vi "Data_base_server.vi"(0 "Raw Data Pathname":path, 1 "Results File Pathname":path, 3 "Clients time":dbl, 4 "Start time":dbl, 5 "End time":dbl, 6 "Average Meas Time (min)":dbl=100.0 format="%.1f", 7 "Channels from Client":string[][](array[string])=[["Data Base:Measurement:Type", "LDA & Cw"], ["Data Base:Position:No of Inst", "2"], ["Data Base:Position:X1", "-60"], ["Data Base:Position:X2", ""], ["Data Base:Position:Y1", "2"], ["Data Base:Position:Y2", "0.00"], ["Data Base:Position:Z1", "0.00"], ["Data Base:Position:Z2", "2.00"]], 8 "Average Sampling freq":sgl=100.0 format="%.1f", 9 "Rig Name":string) -> (14 "Channel names":string[](array[string])=["Data Base:DB:Filename", "Data Base:Start:Date", "Data Base:Start:Time", "EnFlo Tun:Job: Name", "EnFlo Tun:User: Name", "Data Base:Results:Folder", "Data Base:Results:Filename", "Data Base:Measurement:Type", "Data Base:X Axis:Max", "Data Base:X Axis:Min", "Data Base:Y Axis:Max", "Data Base:Y Axis:Min", "Data Base:Z Axis:Max", "Data Base:Z Axis:Min", "Data Base:No of:Measurements", "Data Base:Av Meas:Frequency (Hz)", "Data Base:Av Meas:Time (min)", "EnFlo Tun:labstrat1:Delta T", "EnFlo Tun:Heater Temp:Average", "EnFlo Tun:Inside:Velocity", "EnFlo Tun:Vorticity: Generators", "EnFlo Tun:Barrier Wall: Height", "EnFlo Tun:Roughness: Height", "EnFlo Tun:Side Wall: Separation", "EnFlo Tun:Obstacle/:Building", "EnFlo Tun:Obstacle: Orientation", "GMU:Source: Type", "GMU:Source: Height", "GMU:Release: Orientation", "GMU:Source:Meas Q", "GMU:Source:Meas Strength", "GMU:Trace: Gas", "GMU:Carrier: Gas", "GMU:Source:Release Temp", "GMU:Suction:Meas Q"], 15 "Channel values":string[](array[string])=["1999:May_1999:G3_3 HD_00006", "13/5/99", "1:55 pm", "National Power", "Paul Hayden", "BMT", "default", "LDA, Cw", "100.00", "-60.00", "2.00", "0.00", "0.00", "0.00", "10", "100.00", "100.00", "1.42", "26.63", "1.54", "\"7 quarter elipticals, 1 metre tall\"", "150mm", "20mm", "No sidewalls installed", "National Power Building", "30 deg", "D=17.5mm", "150 mm", "Vertical", "", "", "Ethane", "48% N2 in He", "", ""], 17 "spreadsheet string":string)   [LabVIEW 2012]
doc: "This is an example of using features of the VI Server as a client. It shows how you might browse from one or more applications that may be exporting data from one or more data stations. \n\nThe example shows how to query a server for its list of exported VIs, how to get references to the VIs, and how call them with the Call By Reference function."
uses:
  ADAM_Global.vi
  Sub VI's/Exp conditions/EnFlo_Tun_Setup_global.vi
  Anemometry/Anemometry Sub Vis/Globals/Constants_global.vi
panel:
  out "Output Array":string[][](array[string])
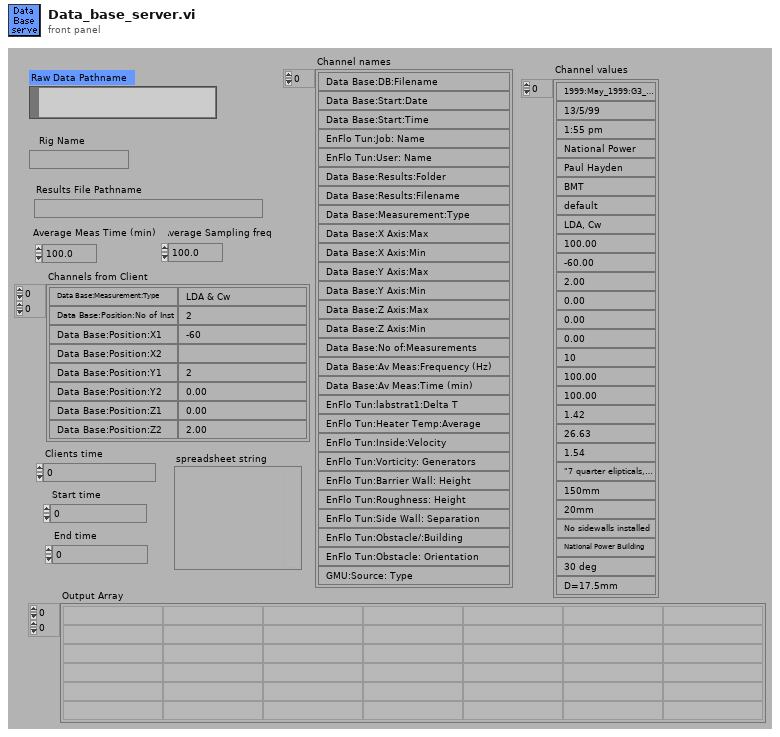
[diagram p1: front panel]
types:
  T1 = cluster{"second":i32, "minute":i32, "hour":i32, "day of month":i32, "month":i32, "year":i32, "day of week":i32, "day of year":i32, "is DST":i32}
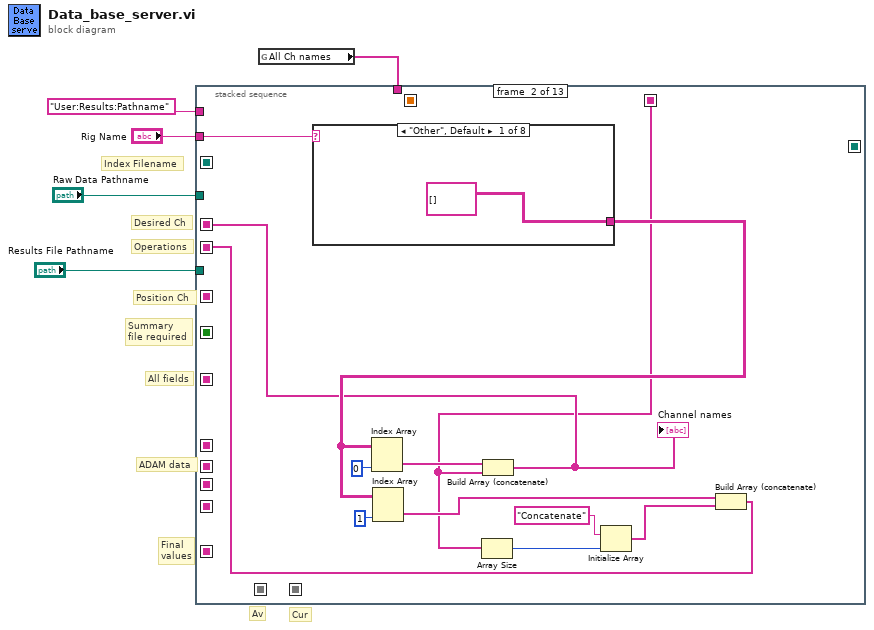
[diagram p0: block diagram]
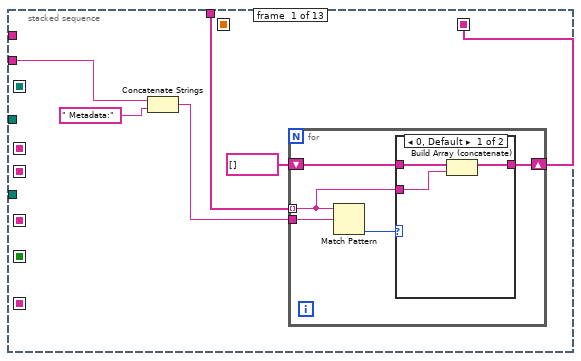
[diagram p2: hidden frame]
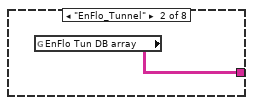
[diagram p4: hidden frame]
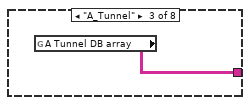
[diagram p5: hidden frame]
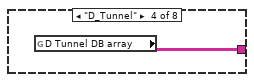
[diagram p6: hidden frame]
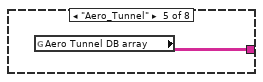
[diagram p7: hidden frame]
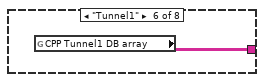
[diagram p8: hidden frame]
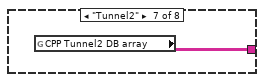
[diagram p9: hidden frame]
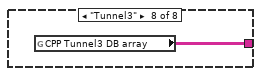
[diagram p10: hidden frame]
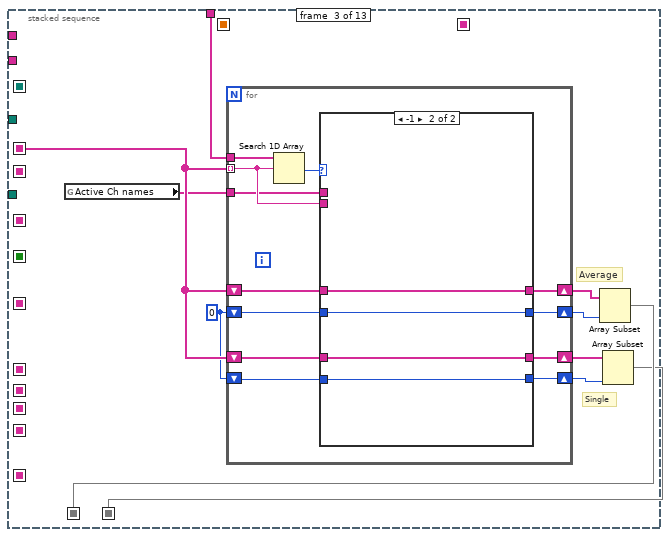
[diagram p11: hidden frame]
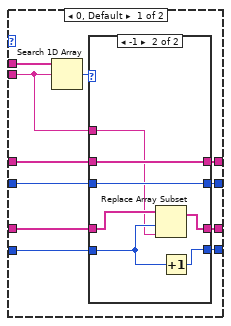
[diagram p12: hidden frame]
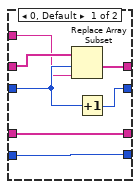
[diagram p13: hidden frame]
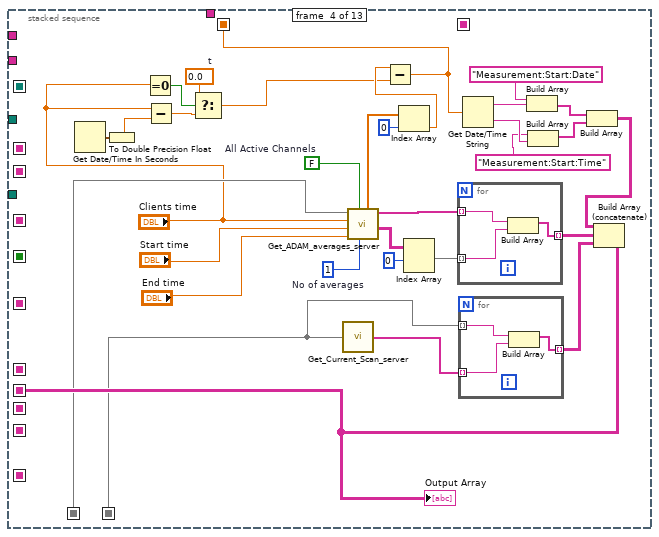
[diagram p14: hidden frame]
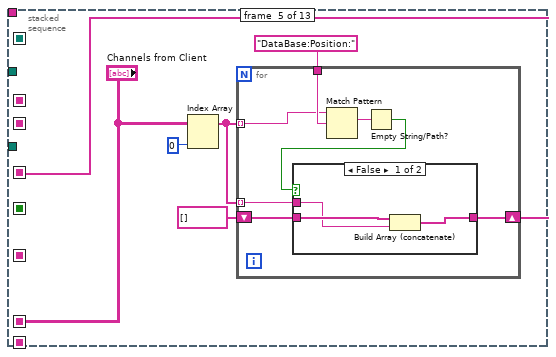
[diagram p15: hidden frame]
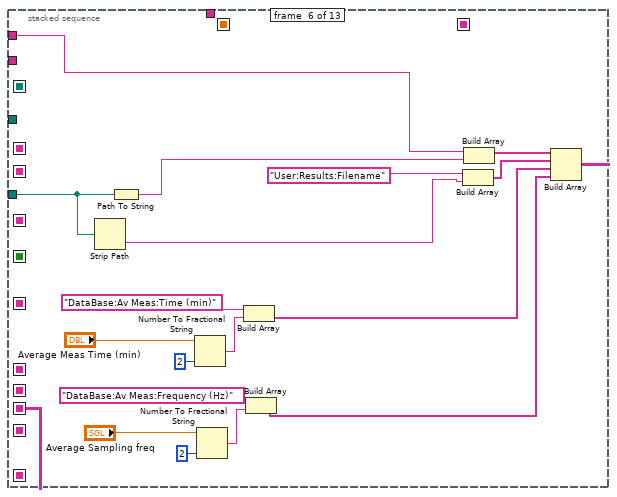
[diagram p17: hidden frame]
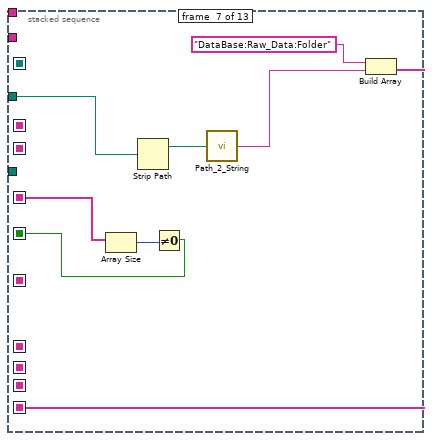
[diagram p18: hidden frame]
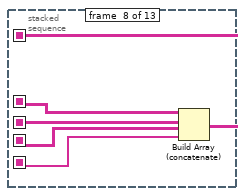
[diagram p19: hidden frame]
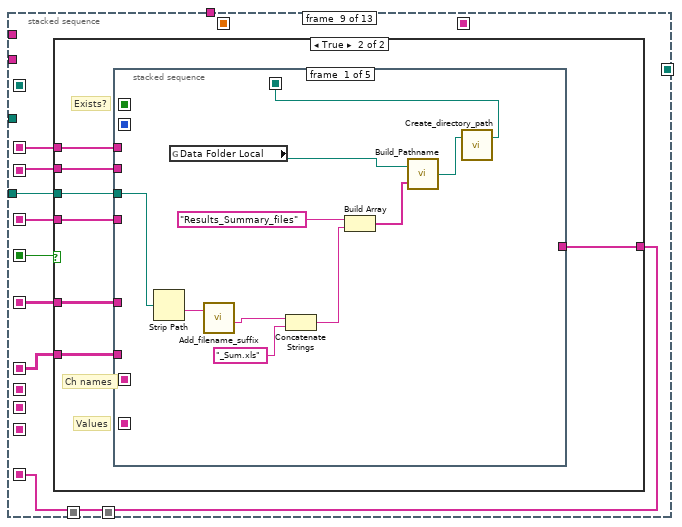
[diagram p20: hidden frame]
diagram:
  # "Cur"
  # "Av"
  # "Index Filename"
  # "Desired Ch"
  # "Operations"
  # "Final\nvalues"
  # "Summary\nfile required"
  # "Position Ch"
  # "All fields"
  # "ADAM data"
  n1 = global read "ADAM_Global.vi" "All Ch names"() -> (w3:string[])
  n2 = stacked-sequence {
    seq-local: [_ w27 _ _ _ _ _ _ _ _ _ _ _] -> [_ _ w50 _ _ _ _ _ w183 _ _ w319 w331]
    seq-local: [_ _ _ w112 _ _ _ _ _ _ _ _ _] -> [_ _ _ _ _ _ _ w177 _ _ _ _ _]
    seq-local: [_ _ _ _ _ w164 _ _ _ _ _ _ _] -> [_ _ _ _ _ _ _ w176 _ _ _ _ _]
    seq-local: [_ _ _ _ _ _ _ w173 _ _ _ _ _] -> [_ _ _ _ _ _ _ _ w181 w280 _ _ _]
    seq-local: [_ _ _ _ _ _ w168 _ _ _ _ _ _] -> [_ _ _ _ _ _ _ w175 _ _ _ _ _]
    seq-local: [_ _ _ _ _ _ _ _ w185 _ _ _ _] -> [_ _ _ _ _ _ _ _ _ w287 _ w320 w330]
    seq-local: [_ _ _ _ w131 _ _ _ _ _ _ _ _] -> [_ _ _ _ _ _ w171 _ w182 _ _ _ _]
    seq-local: [_ _ _ _ "Channels from Client" _ _ _ _ _ _ _ _] -> [_ _ _ _ _ _ _ w174 w178 _ _ _ _]
    seq-local: [_ _ _ _ _ _ w169 _ _ _ _ _ _] -> [_ _ _ _ _ _ _ _ w184 _ _ _ _]
    seq-local: [_ w21 _ _ _ _ _ _ _ _ _ _ _] -> [_ _ _ _ _ _ _ _ w180 _ _ _ _]
    seq-local: [_ _ _ w93 _ _ _ _ _ _ _ _ _] -> [_ _ _ _ _ _ _ _ _ _ _ _ _]
    seq-local: [_ _ _ _ _ _ _ _ _ _ w305 _ _] -> [_ _ _ _ _ _ _ _ _ _ _ w317 w323]
    seq-local: [_ _ w43 _ _ _ _ _ _ _ _ _ _] -> [_ _ _ w104 _ _ _ _ _ _ _ _ _]
    seq-local: [_ _ w42 _ _ _ _ _ _ _ _ _ _] -> [_ _ _ w103 _ _ _ _ _ _ _ _ _]
    seq-local: [w6 _ _ _ _ _ _ _ _ _ _ _ _] -> [_ w24 _ _ _ _ _ _ _ _ _ _ _]
    seq-local: [_ _ _ _ _ _ _ _ _ _ w307 _ _] -> [_ _ _ _ _ _ _ _ _ _ _ _ w322]
    tunnel: "User:Results:Pathname" -> [_ _ _ _ _ w152 _ _ _ _ _ w321 _]
    tunnel: "Results File Pathname" -> [_ _ _ _ _ w149 _ _ w179 _ _ _ _]
    tunnel: "Rig Name" -> [w10 w29 _ _ _ _ _ _ _ w273 w314 _ _]
    tunnel: w3 -> [w8 _ w41 _ _ _ _ _ _ _ _ _ _]
    tunnel: "Raw Data Pathname" -> [_ _ _ _ _ _ w167 _ _ _ _ _ _]
    frame #0 {
      n3 = Concatenate Strings(w10, " Metadata:") -> (w9:string)
      n4 = for {
        tunnel: w9 -> [w13]
        shift-right: [w14] -> w6
        shift-left: string[] [] -> [w15]
        tunnel: w8 -> [w12] mode=indexing
        n5 = Match Pattern(string=w12, regular expression=w13) -> (offset past match=w16:i32)  [unwired: 4 out]
        n6 = case shown="0, Default" w16 {
          tunnel: w15 -> [w19 w20]
          tunnel: [w17 w20] -> w14
          tunnel: w12 -> [w18 _]
          frame 0, Default {
            n7 = Build Array (concatenate)(w19, w18) -> (w17:string[])
          }
          frame -1 {
          }
        }
      }
    }
    frame #1 {
      n8 = case shown="\"Other\", Default" w29 {
        tunnel: [string[][] [] ("EnFlo Tun DB array") w34 w35 w36 w37 w38 w39 w40] -> w30
        frame "Other", Default {
        }
        frame "EnFlo_Tunnel" {
          n9 = global read "EnFlo_Tun_Setup_global.vi" "EnFlo Tun DB array"() -> (w34:string[][])
        }
        frame "A_Tunnel" {
          n10 = global read "EnFlo_Tun_Setup_global.vi" "A Tunnel DB array"() -> (w35:string[][])
        }
        frame "D_Tunnel" {
          n11 = global read "EnFlo_Tun_Setup_global.vi" "D Tunnel DB array"() -> (w36:string[][])
        }
        frame "Aero_Tunnel" {
          n12 = global read "EnFlo_Tun_Setup_global.vi" "Aero Tunnel DB array"() -> (w37:string[][])
        }
        frame "Tunnel1" {
          n13 = global read "EnFlo_Tun_Setup_global.vi" "CPP Tunnel1 DB array"() -> (w38:string[][])
        }
        frame "Tunnel2" {
          n14 = global read "EnFlo_Tun_Setup_global.vi" "CPP Tunnel2 DB array"() -> (w39:string[][])
        }
        frame "Tunnel3" {
          n15 = global read "EnFlo_Tun_Setup_global.vi" "CPP Tunnel3 DB array"() -> (w40:string[][])
        }
      }
      n16 = Index Array(array=w30, index (col)=0) -> (element=w28:string[])  [unwired: 1 in]
      n17 = Index Array(array=w30, index (col)=1) -> (element=w26:string[])  [unwired: 1 in]
      n18 = Array Size(array=w24) -> (size(s)=w25:i32)
      n19 = Build Array (concatenate)(w28, w24) -> (w27:string[])
      "Channel names" <- w27
      n20 = Initialize Array("Concatenate", w25) -> (w22:string[])
      n21 = Build Array (concatenate)(w26, w22) -> (w21:string[])
    }
    frame #2 {
      w48 = 0
      # "Single"
      # "Average"
      n22 = global read "ADAM_Global.vi" "Active Ch names"() -> (w49:string[])
      n23 = for {
        tunnel: w50 -> [w56] mode=indexing
        tunnel: w41 -> [w62]
        shift-right: [w60] -> w47
        shift-left: w50 -> [w59]
        shift-right: [w58] -> w45
        shift-left: w50 -> [w57]
        tunnel: w49 -> [w55]
        shift-right: [w51] -> w46
        shift-left: w48 -> [w52]
        shift-right: [w53] -> w44
        shift-left: w48 -> [w54]
        n24 = Search 1D Array(1D array=w62, element=w56) -> (index of element=w61:i32)  [unwired: 1 out]
        n25 = case shown="-1" w61 {
          tunnel: [w64 w91] -> w60
          tunnel: w59 -> [w65 w91]
          tunnel: [w70 w90] -> w58
          tunnel: w57 -> [w71 w90]
          tunnel: w56 -> [w63 _]
          tunnel: w55 -> [w73 _]
          tunnel: w54 -> [w69 w88]
          tunnel: [w68 w88] -> w53
          tunnel: w52 -> [w67 w89]
          tunnel: [w66 w89] -> w51
          frame 0, Default {
            n26 = Search 1D Array(1D array=w73, element=w63) -> (index of element=w72:i32)  [unwired: 1 out]
            n27 = case shown="-1" w72 {
              tunnel: w71 -> [w76 w87]
              tunnel: [w76 w86] -> w70
              tunnel: w69 -> [w75 w85]
              tunnel: [w75 w84] -> w68
              tunnel: w67 -> [w80 w83]
              tunnel: [w77 w83] -> w66
              tunnel: w65 -> [w79 w82]
              tunnel: [w78 w82] -> w64
              tunnel: w63 -> [w74 w81]
              frame 0, Default {
                n28 = Replace Array Subset(array=w79, new element=w74, index=w80) -> (w78:string[])
                n29 = Increment(x=w80) -> (x+1=w77:i32)
              }
              frame -1 {
                n30 = Replace Array Subset(array=w87, new element=w81, index=w85) -> (w86:string[])
                n31 = Increment(x=w85) -> (x+1=w84:i32)
              }
            }
          }
          frame -1 {
          }
        }
      }
      n32 = Array Subset(array=w47, length=w46) -> (w43:string[])  [unwired: 1 in]
      n33 = Array Subset(array=w45, length=w44) -> (w42:string[])  [unwired: 1 in]
    }
    frame #3 {
      w97 = 0.0  # t
      w105 = FALSE  # All Active Channels
      w123 = 1  # No of averages
      n34 = Get Date/Time In Seconds() -> (seconds since 1Jan1904=w92:timestamp)
      n35 = To Double Precision Float(number=w92) -> (double precision float=w100:dbl)
      n36 = Equal To 0?(x="Clients time") -> (x = 0?=w98:bool)
      n37 = Subtract(x="Clients time", y=w100) -> (x-y=w99:dbl)
      n38 = Select(t=w97, s=w98, f=w99) -> (s? t:f=w94:dbl)
      n39 = call "Get_Current_Scan_server.vi"("Desired Channels"=w103) -> ("String values"=w102:string[])  [unwired: 2 out]
      n40 = call "Get_ADAM_averages_server.vi"("No of averages"=w123, "All Active Channels"=w105, "End time"="End time", "Start time"="Start time", "Clients time"="Clients time", "ADAM Ch Names"=w104) -> ("Values"=w108:string[][], "Titles"=w111:string[], "Times"=w121:dbl[])  [unwired: 2 out]
      n41 = Index Array(array=w121, index=0) -> (element=w95:dbl)
      n42 = Subtract(x=w95, y=w94) -> (x-y=w93:dbl)
      n43 = Index Array(array=w108, index (row)=0) -> (element=w110:string[])  [unwired: 1 in]
      n44 = for {
        tunnel: w111 -> [w129] mode=indexing
        tunnel: w110 -> [w128] mode=indexing
        tunnel: [w127] -> w113 mode=indexing
        n45 = Build Array(w129, w128) -> (w127:string[])
      }
      n46 = for {
        tunnel: w102 -> [w126] mode=indexing
        tunnel: [w125] -> w101 mode=indexing
        tunnel: w103 -> [w124] mode=indexing
        n47 = Build Array(w124, w126) -> (w125:string[])
      }
      n48 = Get Date/Time String(seconds (now)=w93) -> (date string=w119:string, time string=w118:string)  [unwired: 2 out]
      n49 = Build Array("Measurement:Start:Date", w119) -> (w116:string[])
      n50 = Build Array("Measurement:Start:Time", w118) -> (w115:string[])
      n51 = Build Array(w116, w115) -> (w114:string[][])
      n52 = Build Array (concatenate)(w114, w113, w101) -> (w112:string[][])
      "Output Array" <- w112
    }
    frame #4 {
      n53 = Index Array(array="Channels from Client", index (col)=0) -> (element=w133:string[])  [unwired: 1 in]
      n54 = for {
        tunnel: "DataBase:Position:" ("String to match") -> [w142]
        tunnel: w133 -> [w141] mode=indexing
        shift-right: [w136] -> w131
        shift-left: string[] [] -> [w137]
        tunnel: w133 -> [w138] mode=indexing
        n55 = Match Pattern(string=w141, regular expression=w142) -> (match substring=w140:string)  [unwired: 4 out]
        n56 = Empty String/Path?(string/path=w140) -> (empty?=w139:bool)
        n57 = case shown="False" w139 {
          tunnel: w138 -> [w143 _]
          tunnel: w137 -> [w145 w146]
          tunnel: [w144 w146] -> w136
          frame False {
            n58 = Build Array (concatenate)(w145, w143) -> (w144:string[])
          }
          frame True {
          }
        }
      }
    }
    frame #5 {
      n59 = Strip Path(path=w149) -> (name=w148:string)  [unwired: 1 out]
      n60 = Path To String(path=w149) -> (string=w151:string)
      n61 = Number To Fractional String(number="Average Meas Time (min)", precision (6)=i16 2) -> (F-format string=w161:string)  [unwired: 2 out]
      n62 = Number To Fractional String(number="Average Sampling freq", precision (6)=i16 2) -> (F-format string=w159:string)  [unwired: 2 out]
      n63 = Build Array("DataBase:Av Meas:Time (min)", w161) -> (w155:string[])
      n64 = Build Array("DataBase:Av Meas:Frequency (Hz)", w159) -> (w154:string[])
      n65 = Build Array("User:Results:Filename", w148) -> (w147:string[])
      n66 = Build Array(w152, w151) -> (w153:string[])
      n67 = Build Array(w153, w147, w155, w154) -> (w164:string[][])
    }
    frame #6 {
      n68 = Array Size(array=w171) -> (size(s)=w170:i32)
      n69 = Strip Path(path=w167) -> (stripped path=w166:path)  [unwired: 1 out]
      n70 = Not Equal To 0?(x=w170) -> (x != 0?=w169:bool)
      n71 = call "Path_2_String.vi"("Real Path"=w166) -> ("Path String"=w165:string)
      n72 = Build Array("DataBase:Raw_Data:Folder", w165) -> (w168:string[])
    }
    frame #7 {
      n73 = Build Array (concatenate)(w174, w177, w176, w175) -> (w173:string[][])
    }
    frame #8 {
      n74 = case shown="True" w184 {
        tunnel: [w187 w199] -> w185
        tunnel: w183 -> [w188 w198]
        tunnel: w182 -> [_ w197]
        tunnel: w181 -> [w189 w196]
        tunnel: w180 -> [_ w195]
        tunnel: w179 -> [_ w194]
        tunnel: w178 -> [_ w193]
        frame False {
          n75 = Index Array(array=w189, index (col)=1) -> (element=w190:string[])  [unwired: 1 in]
          n76 = Index Array(array=w189, index (col)=0) -> (element=w186:string[])  [unwired: 1 in]
          n77 = call "Merge_row_values.vi"("Present Row values"=w190, "Present Channels"=w186, "Desired Channels"=w188) -> ("Desired Row values"=w187:string[])  [unwired: 1 out]
        }
        frame True {
          # "Exists?"
          # "Ch names"
          # "Values"
          n78 = stacked-sequence {
            seq-local: [_ _ w230 _ _] -> [_ _ _ w246 w269]
            seq-local: [_ _ w226 _ _] -> [_ _ _ w250 w271]
            seq-local: [w207 _ _ _ _] -> [_ w213 w228 _ w272]
            seq-local: [_ w210 _ _ _] -> [_ _ w222 _ w270]
            seq-local: [_ _ w223 _ _] -> [_ _ _ _ w268]
            tunnel: [_ _ _ w251 _] -> w199
            tunnel: w198 -> [_ _ w229 w248 _]
            tunnel: w197 -> [_ _ w236 _ _]
            tunnel: w196 -> [_ _ w232 _ _]
            tunnel: w195 -> [_ _ _ w249 _]
            tunnel: w194 -> [w208 _ _ _ _]
            tunnel: w193 -> [_ w216 _ _ _]
            frame #0 {
              n79 = Strip Path(path=w208) -> (name=w201:string)  [unwired: 1 out]
              n80 = global read "Constants_global.vi" "Data Folder Local"() -> (w206:path)
              n81 = call "Add_filename_suffix.vi"("Filename"=w201) -> ("Base name"=w200:string)  [unwired: 1 in, 3 out]
              n82 = Concatenate Strings(w200, "_Sum.xls" ("Substring")) -> (w202:string)
              n83 = Build Array("Results_Summary_files", w202) -> (w205:string[])
              n84 = call "Build_Pathname.vi"("PathElements"=w205, "PathnameIn"=w206) -> ("AppendedPath"=w203:path)
              n85 = call "Create_directory_path.vi"("Path name"=w203) -> ("Path name Out"=w207:path)  [unwired: 1 in, 1 out]
            }
            frame #1 {
              n86 = Index Array(array=w216, index (col)=0) -> (element=w220:string[])  [unwired: 1 in]
              n87 = Search 1D Array(1D array=w220, element="Does the results file already exist?") -> (index of element=w217:i32)  [unwired: 1 out]
              n88 = Index Array(array=w216, index (row)=w217, index (col)=1 ("Index")) -> (element=w215:string)
              n89 = call "Does_file_exist_(simple).vi"("Pathname"=w213) -> ("exists?"=w211:bool)
              n90 = Not Equal?(x="FALSE", y=w215) -> (x != y?=w212:bool)
              n91 = And(x=w211, y=w212) -> (x .and. y?=w210:bool)
            }
            frame #2 {
              n92 = Build Array (concatenate)(w229, w236) -> (w235:string[])
              n93 = case shown="True" w222 {
                tunnel: w235 -> [w239 w245]
                tunnel: w228 -> [_ w244]
                tunnel: [w239 w243] -> w226
                tunnel: [string[][] [] ("Channel Values") w242] -> w224
                tunnel: [0 ("Offset from File End") w241] -> w223
                frame False {
                }
                frame True {
                  n94 = call "Read_Ch_data_file.vi"("Present Channels"=w245, "Output"=enum16{"All Ch data", "The last few rows"}."All Ch data", "Filename"=w244) -> ("Channel Values"=w242:string[][], "Merged Channels"=w243:string[], "Offset from File End"=w241:i32)  [unwired: 2 in, 2 out]
                }
              }
              n95 = Index Array(array=w232, index (col)=1) -> (element=w231:string[])  [unwired: 1 in]
              n96 = Index Array(array=w232, index (col)=0) -> (element=w227:string[])  [unwired: 1 in]
              n97 = call "Merge_row_values.vi"("Present Row values"=w231, "Present Channels"=w227, "Desired Channels"=w226) -> ("Desired Row values"=w225:string[])  [unwired: 1 out]
              n98 = Build Array (concatenate)(w224, w225) -> (w230:string[][])
            }
            frame #3 {
              n99 = call "Average_Column_Values.vi"("Present Values"=w246, "Present Channels"=w250, "Channel operations"=w249, "Channel names for operations"=w248) -> ("Desired Row values"=w247:string[])
              n100 = call "String_to_Pos_array.vi"("Channel values"=w246, "Channel names"=w250) -> ("Positions"=w254:dbl[][], "No of Inst"=w253:i32)
              n101 = while {
                tunnel: [w260] -> w252
                tunnel: w253 -> [w264]
                tunnel: w254 -> [w259]
                i -> [w257]
                stop <- w261 continue-if-true
                w255 = 3 ("x")
                n102 = Increment(x=w257) -> (x+1=w265:i32)
                n103 = Multiply(x=w255, y=w257) -> (x*y=w256:i32)
                n104 = Array Subset(array=w259, index (col)=w256, length (col)=w255) -> (w258:dbl[][])  [unwired: 2 in]
                n105 = call "Cal_Pos_Max_Min.vi"("Positions"=w258) -> ("Position Info"=w260:string[][], "Instrument moved?"=w262:bool)
                n106 = Less?(x=w265, y=w264) -> (x < y?=w263:bool)
                n107 = Compound Arithmetic op=AND(invert w262, w263) -> (w261:bool)
              }
              n108 = call "Replace_Channel_Values.vi"("Channels to replace"=w252, "Present Values"=w247, "Present Channels"=w248) -> ("Merged Row values"=w251:string[])  [unwired: 1 out]
            }
            frame #4 {
              w266 = TRUE  # Lock File
              w267 = TRUE  # Append last row only
              n109 = call "Write_Ch_data_file.vi"("Append last row only"=w267, "Lock File"=w266, "exists?"=w270, "Write offset fr file end"=w268, "Channel Values"=w269, "Channel names"=w271, "Filename"=w272) -> ()  [unwired: 1 in, 4 out]
            }
          }
        }
      }
    }
    frame #9 {
      n110 = Index Array(array=w280, index (col)=0) -> (element=w284:string[])  [unwired: 1 in]
      n111 = Concatenate Strings(w273, ":Pitot:Velocity" ("Substring")) -> (w286:string)
      n112 = Concatenate Strings(w273, ":Speed:Dem Velocity" ("Substring")) -> (w275:string)
      n113 = Concatenate Strings(w273, ":Speed:Calib Tweak" ("Substring")) -> (w274:string)
      n114 = Build Array(w275, w274, w286) -> (w283:string[])
      n115 = for {
        tunnel: w284 -> [w303]
        tunnel: w283 -> [w302] mode=indexing
        tunnel: [w301] -> w282 mode=indexing
        tunnel: [w300] -> w279 mode=indexing
        n116 = Search 1D Array(1D array=w303, element=w302) -> (index of element=w300:i32)  [unwired: 1 out]
        n117 = Greater Or Equal To 0?(x=w300) -> (x >= 0?=w301:bool)
      }
      n118 = And Array Elements(Boolean array=w282) -> (logical AND=w281:bool)
      n119 = case shown="True" w281 {
        tunnel: w280 -> [_ w294]
        tunnel: w279 -> [_ w292]
        tunnel: w273 -> [_ w290]
        frame False {
        }
        frame True {
          w288 = FALSE  # Tunnel Heated?
          n120 = Index Array(array=w294, index (col)=1) -> (element=w293:string[])  [unwired: 1 in]
          n121 = for {
            tunnel: w293 -> [w299]
            tunnel: w292 -> [w298] mode=indexing
            tunnel: [w296] -> w291 mode=indexing
            n122 = Index Array(array=w299, index=w298) -> (element=w297:string)
            n123 = Fract/Exp String To Number(string=w297) -> (number=w296:dbl)  [unwired: 4 out]
          }
          n124 = call "Add_to_speed_calib_file.vi"("New Row"=w291, "Tunnel Heated?"=w288, "Rig Name"=w290, "Mode"=enum16{"Add Row", "Get Error Value"}."Add Row") -> ()  [unwired: 2 in, 2 out]
        }
      }
      "Channel values" <- w287
    }
    frame #10 {
      n125 = Get Date/Time In Seconds() -> (seconds since 1Jan1904=w304:timestamp)
      n126 = global read "Constants_global.vi" "Data Folder Local"() -> (w309:path)
      n127 = call <vilib>:"LV70TimeStampToDateRec.vi"("time stamp"=w304) -> ("date time rec"=w316:T1)
      n128 = global read "Constants_global.vi" "Data Folder"() -> (w308:path)
      n129 = Unbundle By Name(w316) -> ("year"=w315:i32)
      n130 = Number To Decimal String(number=w315) -> (decimal integer string=w311:string)  [unwired: 1 out]
      n131 = Format Into String(format string="-%s.xls", initial string=w314, w311) -> (resulting string=w313:string)  [unwired: 1 in, 1 out]
      n132 = Build Array(w311, w314, w313) -> (w310:string[])
      n133 = call "Build_Pathname.vi"("PathElements"=w310, "PathnameIn"=w308) -> ("AppendedPath"=w307:path)
      n134 = call "Build_Pathname.vi"("PathElements"=w310, "PathnameIn"=w309) -> ("AppendedPath"=w306:path)
      n135 = call "Create_directory_path.vi"("Path name"=w306) -> ("Path name Out"=w305:path)  [unwired: 1 in, 1 out]
    }
    frame #11 {
      n136 = call "Update_Ch_data_file.vi"("Range"=enum16{"All Ch data", "The last few rows"}."The last few rows", "Channel to search on"=w321, "New Row values"=w320, "Present Channels"=w319, "Filename"=w317) -> ()  [unwired: 2 in, 5 out]
    }
    frame #12 {
      w332 = string[] []
      n137 = for {
        shift-right: [w341] -> w325
        shift-left: w332 -> [w342]
        shift-right: [w343] -> w329
        shift-left: w332 -> [w344]
        tunnel: w330 -> [w340] mode=indexing
        tunnel: w331 -> [w339] mode=indexing
        n138 = Empty String/Path?(string/path=w340) -> (empty?=w345:bool)
        n139 = case shown="True" w345 {
          tunnel: w344 -> [w351 w353]
          tunnel: [w350 w353] -> w343
          tunnel: w342 -> [w349 w352]
          tunnel: [w348 w352] -> w341
          tunnel: w340 -> [w347 _]
          tunnel: w339 -> [w346 _]
          frame False {
            n140 = Build Array (concatenate)(w351, w346) -> (w350:string[])
            n141 = Build Array (concatenate)(w349, w347) -> (w348:string[])
          }
          frame True {
          }
        }
      }
      n142 = for {
        tunnel: w329 -> [w338] mode=indexing
        tunnel: [w337] -> w328 mode=indexing
        tunnel: [w336] -> w327 mode=indexing
        tunnel: [w335] -> w326 mode=indexing
        n143 = call "Split_Ch_name.vi"("Ch name"=w338) -> ("Top level"=w337:string, "Middle"=w336:string, "Low level"=w335:string)
      }
      n144 = call "Updated_File_Copy.vi"("Target Path"=w322, "Source Path"=w323) -> ()  [unwired: 2 out]
      n145 = Build Array(w328, w327, w326, w325) -> (w324:string[][])
      n146 = Array To Spreadsheet String(array=w324, 3:"%s" ("format string")) -> (spreadsheet string=→"spreadsheet string":string)  [unwired: 1 out]
    }
  }
